vi "Gen Field Filter Statement.vi"(10 "Fields Info":T1[](array[typedef]), 11 "Cluster Items in":T3[](array[typedef])) -> (3 "Cluster Items out":T3[](array[typedef]))   [LabVIEW 2021]
uses:
  vi_script.lib/Cluster Item Info.ctl
  <vilib>/Utility/Data Type/Type Definitions/Data Type.ctl
  SQLite Field Info.ctl
  SQLite Data Type.ctl
  SQL-LV/src/db_script/SQLite Data Type to LV Data Type.ctl
  <vilib>/Utility/Data Type/NI_Data Type.lvlib
  EDT SQLite+.lvlib
  vi_script.lib/EDT VI Script.lvlib
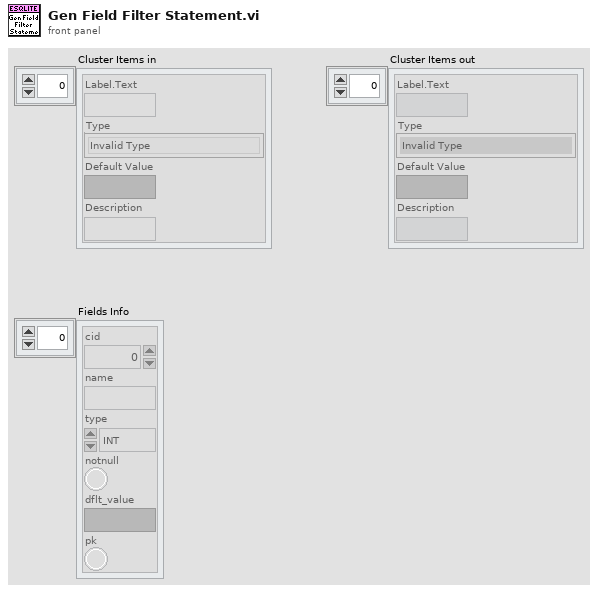
[diagram p1: front panel]
types:
  T1 = typedef "EDT SQLite+.lvlib/SQLite Field Info.ctl" = cluster{"cid":i32, "name":string, "type":T2, "notnull":bool, "dflt_value":variant, "pk":bool}
  T2 = typedef "EDT SQLite+.lvlib/SQLite Data Type.ctl" = enum16{"INT", "INTEGER", "TINYINT", "SMALLINT", "MEDIUMINT", "BIGINT", "UNSIGNED BIG INT", "INT2", "INT8", "CHARACTER", "VARCHAR", "VARYING CHARACTER", "NCHAR", "NATIVE CHARACTER", "NVARCHAR", "TEXT", "CLOB", "BLOB", "no datatype specified", "REAL", "DOUBLE", "DOUBLE PRECISION", "FLOAT", "NUMERIC", "DECIMAL", "BOOLEAN", "DATE", "DATETIME"}
  T3 = typedef "EDT VI Script.lvlib/Cluster Item Info.ctl" = cluster{"Label.Text":string, "Type":T4, "Default Value":variant, "Description":string}
  T4 = typedef "NI_Data Type.lvlib/Data Type.ctl" = enum8{"Invalid Type", "Void", "I8", "I16", "I32", "I64", "U8", "U16", "U32", "U64", "Single Float", "Double Float", "Extended Float", "Single Complex", "Double Complex", "Extended Complex", "Enum U8", "Enum U16", "Enum U32", "Enum U64", "Single Float With Unit", "Double Float With Unit", "Extended Float With Unit", "Single Complex with Unit", "Double Complex with Unit", "Extended Complex with Unit", "Boolean", "String", "Path", "Picture", "Tag", "Array", "Cluster", "Variant", "LV Variant", "Waveform", "Timestamp", "Digital Waveform", "Digital Data", "ExpressData", "Refnum", "External Data", "VI", "Poly VI", "LabVIEW Class Instance", "Fixed Point", "Set Collection", "Map Collection"}
  T5 = typedef "SQLite Data Type to LV Data Type.ctl" = map{T2, T4}
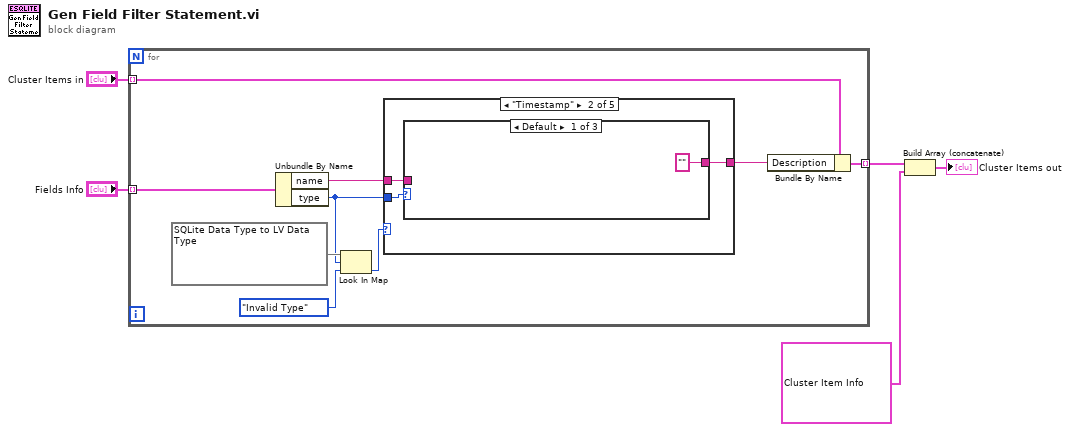
[diagram p0: block diagram]
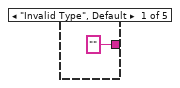
[diagram p2: hidden frame]
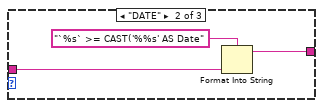
[diagram p3: hidden frame]
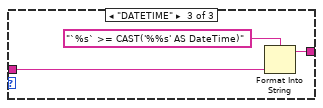
[diagram p4: hidden frame]
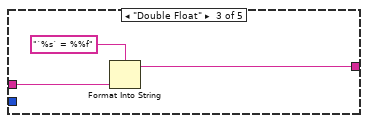
[diagram p5: hidden frame]
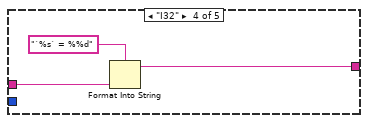
[diagram p6: hidden frame]
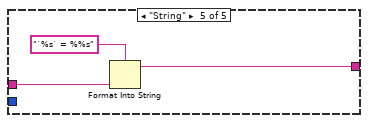
[diagram p7: hidden frame]
diagram:
  n1 = for {
    tunnel: "Cluster Items in" -> [w14] mode=indexing
    tunnel: "Fields Info" -> [w12] mode=indexing
    tunnel: [w13] -> w3 mode=indexing
    n2 = Unbundle By Name(w12) -> ("name"=w8:string, "type"=w6:T2)
    n3 = Look In Map(map=T5 {enum."INT"=enum."I32", enum."INTEGER"=enum."I32", enum."TINYINT"=enum."I32", enum."SMALLINT"=enum."I32", enum."MEDIUMINT"=enum."I32", enum."BIGINT"=enum."I32", enum."UNSIGNED BIG INT"=enum."I32", enum."INT2"=enum."I32", enum."INT8"=enum."I32", enum."CHARACTER"=enum."String", enum."VARCHAR"=enum."String", enum."VARYING CHARACTER"=enum."String", enum."NCHAR"=enum."String", enum."NATIVE CHARACTER"=enum."String", enum."NVARCHAR"=enum."String", enum."TEXT"=enum."String", enum."CLOB"=enum."String", enum."BLOB"=enum."String", enum."no datatype specified"=enum."String", enum."REAL"=enum."Double Float", enum."DOUBLE"=enum."Double Float", enum."DOUBLE PRECISION"=enum."Double Float", enum."FLOAT"=enum."Double Float", enum."NUMERIC"=enum."Double Float", enum."DECIMAL"=enum."Double Float", enum."BOOLEAN"=enum."I32", enum."DATE"=enum."Timestamp", enum."DATETIME"=enum."Timestamp"} ("SQLite Data Type to LV Data Type"), key=w6, default value=Data_Type."Invalid Type" ("type")) -> (value=w9:T4)  [unwired: 1 out]
    n4 = case shown="\"Timestamp\"" w9 {
      tunnel: w8 -> [_ w16 w27 w30 w33]
      tunnel: ["" ("name") w17 w26 w29 w32] -> w7
      tunnel: w6 -> [_ w18 _ _ _]
      frame "Invalid Type", Default {
      }
      frame "Timestamp" {
        n5 = case shown="Default" w18 {
          tunnel: ["" w20 w24] -> w17
          tunnel: w16 -> [_ w21 w23]
          frame Default {
          }
          frame "DATE" {
            n6 = Format Into String(format string="`%s` >= CAST('%%s' AS Date", w21) -> (resulting string=w20:string)  [unwired: 2 in, 1 out]
          }
          frame "DATETIME" {
            n7 = Format Into String(format string="`%s` >= CAST('%%s' AS DateTime)", w23) -> (resulting string=w24:string)  [unwired: 2 in, 1 out]
          }
        }
      }
      frame "Double Float" {
        n8 = Format Into String(format string="`%s` = %%f", w27) -> (resulting string=w26:string)  [unwired: 2 in, 1 out]
      }
      frame "I32" {
        n9 = Format Into String(format string="`%s` = %%d", w30) -> (resulting string=w29:string)  [unwired: 2 in, 1 out]
      }
      frame "String" {
        n10 = Format Into String(format string="`%s` = %%s", w33) -> (resulting string=w32:string)  [unwired: 2 in, 1 out]
      }
    }
    n11 = Bundle By Name(cluster=w14, "Description"=w7) -> (w13:T3)
  }
  n12 = Build Array (concatenate)(w3, T3 {"Label.Text"="Search", "Type"=enum."String", "Default Value"=variant(string ""), "Description"="%+% Like '%%s%'"} ("Cluster Item")) -> (→"Cluster Items out":T3[])
